vi "FTW-JSON-LexicalScan-String.vi"(0 "JSON String":T1, 11 "error in":errorcluster) -> (4 "JSON String Out":T1, 8 "String":string, 15 "error out":errorcluster)   [LabVIEW 2015]
uses:
  FTW-JSON-LexicalScan.ctl
panel:
  # "Inputs"
  # "Outputs"
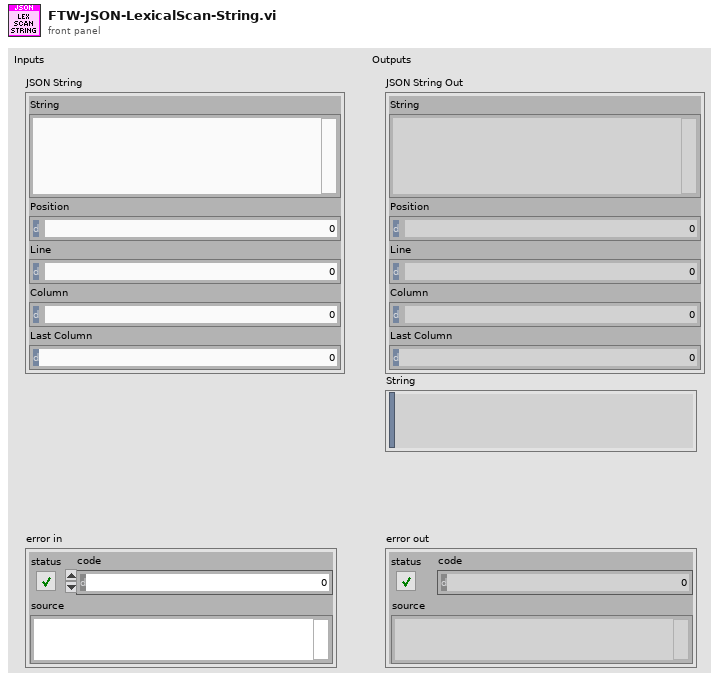
[diagram p1: front panel]
types:
  T1 = typedef "FTW-JSON-LexicalScan.ctl" = cluster{"String":string, "Position":i32, "Line":i32, "Column":i32, "Last Column":i32}
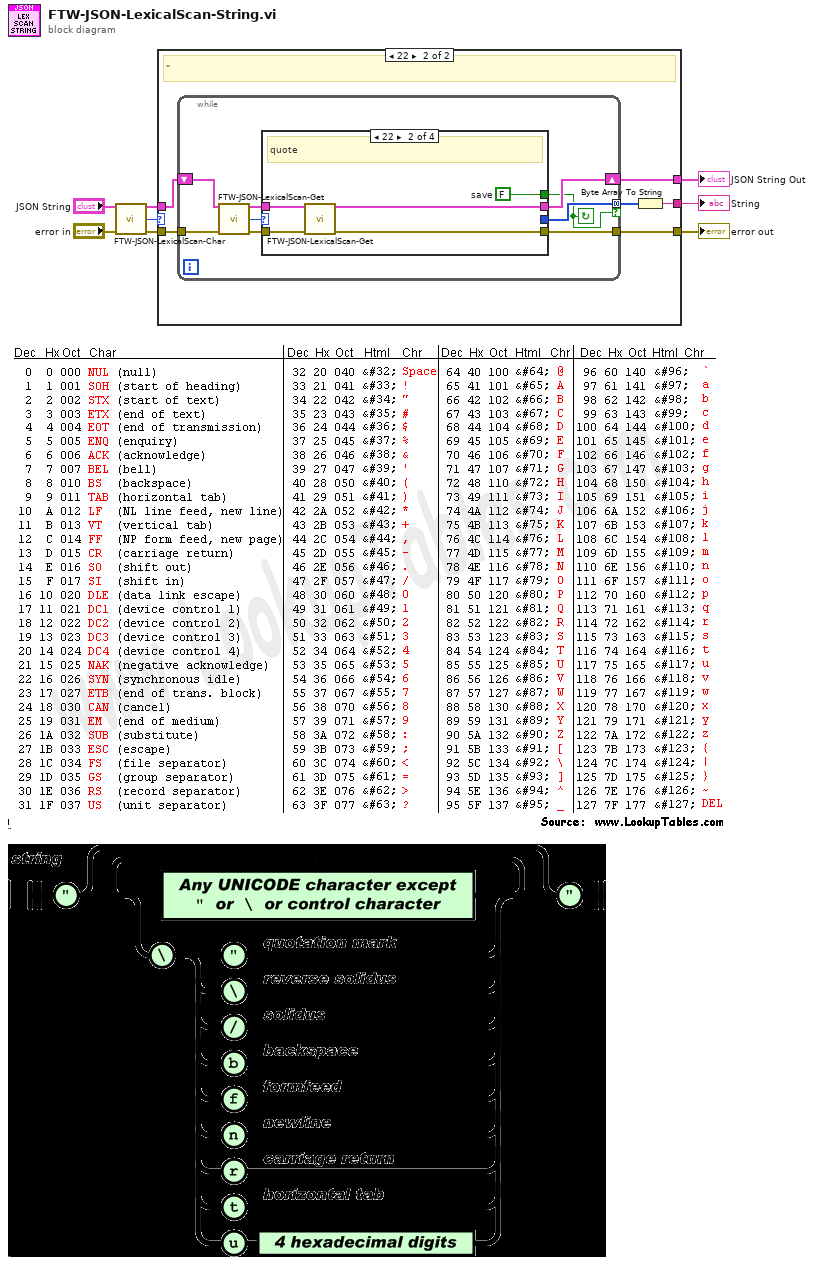
[diagram p0: block diagram]
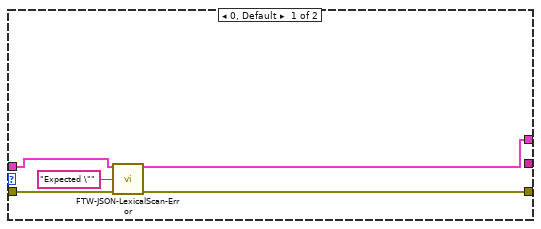
[diagram p2: hidden frame]
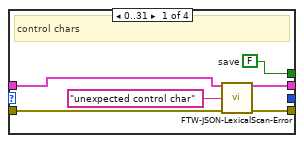
[diagram p3: hidden frame]
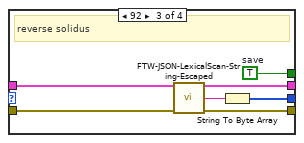
[diagram p4: hidden frame]
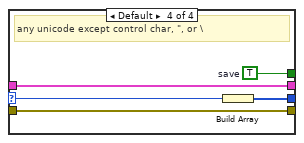
[diagram p5: hidden frame]
diagram:
  n1 = call "FTW-JSON-LexicalScan-Char.vi"("JSON String"="JSON String", "error in"="error in") -> ("JSON String Out"=w2:T1, "Char"=w1:u8, "error out"=w3:errorcluster)  [unwired: 11 in]
  n2 = case shown="22" w1 {
    tunnel: [w10 w19] -> w7
    tunnel: [_ w17] -> w6
    tunnel: [w9 w16] -> w4
    tunnel: w3 -> [w11 w15]
    tunnel: w2 -> [w12 w14]
    frame 0, Default {
      n3 = call "FTW-JSON-LexicalScan-Error.vi"("JSON String"=w12, "Error String"="Expected \"" ("Error Message"), "error in"=w11) -> ("JSON String Out"=w9:T1, "error out"=w10:errorcluster)  [unwired: 11 in]
    }
    frame 34 {
      # "\""
      n4 = while {
        shift-right: [w26] -> w16
        shift-left: w14 -> [w25]
        tunnel: w15 -> [w24]
        tunnel: [w28] -> w19
        tunnel: [w27] -> w18 mode=concatenating if=w20
        stop <- w20 continue-if-true
        n5 = call "FTW-JSON-LexicalScan-Get.vi"("JSON String"=w25, "error in"=w24) -> ("JSON String Out"=w22:T1, "Char"=w21:u8, "error out"=w23:errorcluster)  [unwired: 11 in]
        n6 = case shown="22" w21 {
          selector: w21 -> [_ _ _ w50]
          tunnel: w22 -> [w31 w37 w41 w47]
          tunnel: w23 -> [w34 w39 w46 w51]
          tunnel: [w32 w38 w45 w51] -> w28
          tunnel: [_ _ w43 w48] -> w27
          tunnel: [w33 w35 w42 w49] -> w20
          tunnel: [w30 w36 w40 w47] -> w26
          frame 0..31 {
            w33 = FALSE  # save
            # "control chars"
            n7 = call "FTW-JSON-LexicalScan-Error.vi"("JSON String"=w31, "Error String"="unexpected control char", "error in"=w34) -> ("JSON String Out"=w30:T1, "error out"=w32:errorcluster)  [unwired: 11 in]
          }
          frame 34 {
            w35 = FALSE  # save
            # "quote"
            n8 = call "FTW-JSON-LexicalScan-Get.vi"("JSON String"=w37, "error in"=w39) -> ("JSON String Out"=w36:T1, "error out"=w38:errorcluster)  [unwired: 11 in, 1 out]
          }
          frame 92 {
            w42 = TRUE  # save
            # "reverse solidus"
            n9 = call "FTW-JSON-LexicalScan-String-Escaped.vi"("JSON String"=w41, "error in"=w46) -> ("JSON String Out"=w40:T1, "String"=w44:string, "error out"=w45:errorcluster)  [unwired: 11 in]
            n10 = String To Byte Array(string=w44) -> (unsigned byte array=w43:u8[])
          }
          frame Default {
            w49 = TRUE  # save
            # "any unicode except control char, \", or \\"
            n11 = Build Array(w50) -> (w48:u8[])
          }
        }
      }
      n12 = Byte Array To String(unsigned byte array=w18) -> (string=w17:string)
    }
  }
  "String" <- w6
  "error out" <- w7
  "JSON String Out" <- w4
